vi "VIE.Module.Queued Message Handler.dqClass_Delete.vi"(0 "reference":T2, 3 "timeout in ms (10000)":i32=10000, 5 "error in (no error)":errorcluster) -> (16 "data":T1, 17 "timed out?":bool, 19 "error out":errorcluster)   [LabVIEW 2010, in "VIE.Module.Queued Message Handler.QueuedMessageHandler.dqGOOPClass.lvlib"]
doc: "Deletes the dqGOOP object and releases all refnums associated with the object."
uses:
  VIE.Module.Queued Message Handler.QueuedMessageHandler.dqGOOPClass.lvlib
  VIE.Module.Queued Message Handler.dqClass_ObjectReference.ctl
  VIE.Module.Queued Message Handler.dqClass_ObjectData.ctl
panel:
  in  "queue (default)":refnum<queue>
  # "Copyright (C) 2004 DataAct Incorporated"
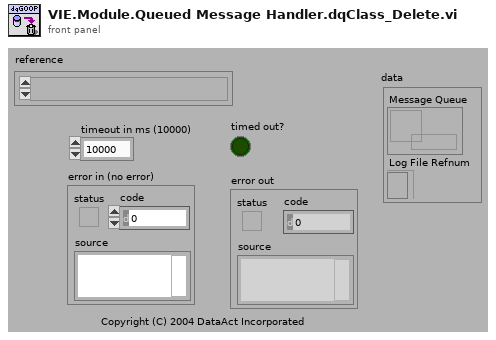
[diagram p1: front panel]
types:
  T1 = typedef "VIE.Module.Queued Message Handler.QueuedMessageHandler.dqGOOPClass.lvlib/VIE.Module.Queued Message Handler.dqClass_ObjectData.ctl" = cluster{"Message Queue":refnum<queue>, "Log File Refnum":refnum<file>}
  T2 = typedef "VIE.Module.Queued Message Handler.QueuedMessageHandler.dqGOOPClass.lvlib/VIE.Module.Queued Message Handler.dqClass_ObjectReference.ctl" = refnum<k1>
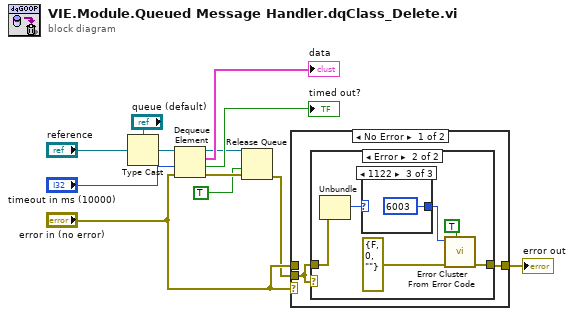
[diagram p0: block diagram]
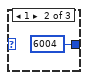
[diagram p4: hidden frame]
diagram:
  n1 = Type Cast(type="queue (default)", x="reference") -> (*(type *) &x=w6:refnum<queue>)
  n2 = Dequeue Element(queue=w6, timeout in ms (-1)="timeout in ms (10000)", error in (no error)="error in (no error)") -> (queue out=w9:refnum<queue>, element=→"data":T1, timed out?=→"timed out?":bool, error out=w8:errorcluster)
  n3 = Release Queue(queue=w9, force destroy? (F)=TRUE, error in (no error)=w8) -> (error out=w2:errorcluster)  [unwired: 2 out]
  n4 = case shown="No Error" "error in (no error)" {
    tunnel: [w13 w25] -> w1
    tunnel: "error in (no error)" -> [_ w25]
    tunnel: w2 -> [w14 _]
    frame No Error {
      n5 = case shown="Error" w14 {
        tunnel: [w15 w16] -> w13
        tunnel: w14 -> [w15 w21]
        frame No Error {
        }
        frame Error {
          n6 = Unbundle(w21) -> ("code"=w20:i32)  [unwired: 2 out]
          n7 = case shown="1122" w20 {
            selector: w20 -> [w22 _ _]
            tunnel: [w22 6004 ("code") 6003 ("code")] -> w18
            frame Default {
            }
            frame 1 {
            }
            frame 1122 {
            }
          }
          n8 = call <vilib>:"Error Cluster From Error Code.vi"("show call chain? (False)"=TRUE, "error in (no error)"=errorcluster {"status"=FALSE, "code"=0, "source"=""} ("error out"), "error code (0)"=w18) -> ("error out"=w16:errorcluster)  [unwired: 6 in]
        }
      }
    }
    frame Error {
    }
  }
  "error out" <- w1
